vi "VI Server_Set ComboBox by Item Selected.vi"(7 "Label":string, 8 "error in":errorcluster, 9 "Item Selected":string, 11 "VI Server Cluster":T1) -> (0 "error out":errorcluster, 1 "ComboBoxRef":refnum<vi>, 3 "VI Server Cluster.DUP":T1)   [LabVIEW 2020, in "VI Server Toolkit LV2013.lvlib"]
doc: "Sets Menu Ring value/selection by the item name."
uses:
  VI Server Toolkit LV2013.lvlib
  VI Server_TypeDefs/VI Server_RefsCluster.ctl
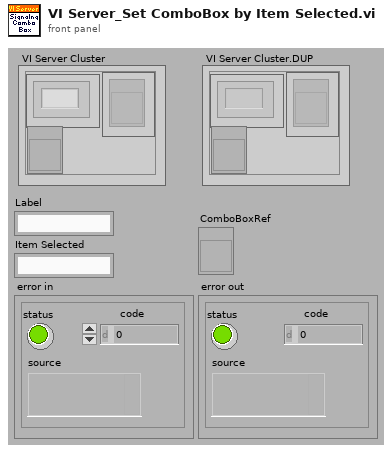
[diagram p1: front panel]
types:
  T1 = typedef "VI Server_RefsCluster.ctl" = cluster{"Labels":string[], "Refs":refnum<vi>[], "VI Ref":refnum<vi>}
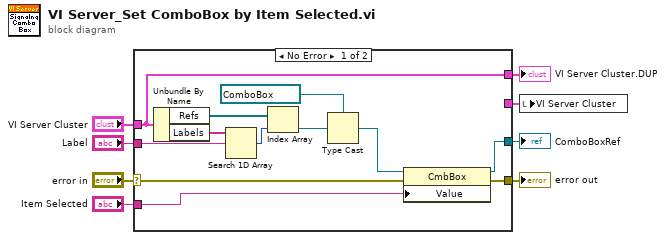
[diagram p0: block diagram]
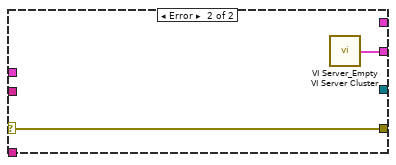
[diagram p2: hidden frame]
diagram:
  n1 = case shown="No Error" "error in" {
    selector: "error in" -> [w12 w22]
    tunnel: "Label" -> [w19 _]
    tunnel: "VI Server Cluster" -> [w9 _]
    tunnel: [w15 w22] -> w8
    tunnel: [w14 _] -> w3
    tunnel: "Item Selected" -> [w10 _]
    tunnel: [w9 _] -> w2
    tunnel: [_ w21] -> w1
    frame No Error {
      n2 = Unbundle By Name(w9) -> ("Refs"=w17:refnum<vi>[], "Labels"=w20:string[])
      n3 = Search 1D Array(1D array=w20, element=w19) -> (index of element=w18:i32)  [unwired: 1 out]
      n4 = Index Array(array=w17, index=w18) -> (element=w16:refnum<vi>)
      n5 = Type Cast(type=refnum<vi> refnum ("Combo Box"), x=w16) -> (*(type *) &x=w11:refnum<vi>)
      n6 = property class="CmbBox"(reference=w11, error in=w12, "Value"=w10) -> (reference out=w14:refnum<vi>, error out=w15:errorcluster)
    }
    frame Error {
      n7 = call "VI Server_Empty VI Server Cluster.vi"() -> ("VI Server Cluster"=w21:T1)  [unwired: 7 in]
    }
  }
  "error out" <- w8
  "VI Server Cluster.DUP" <- w2
  "ComboBoxRef" <- w3
  n8 = local write "VI Server Cluster"(w1) -> ()
